vi "Read Available Data Names.vi"(8 "error in (no error)":errorcluster, 11 "ControlDropMsg in":refnum<class "ControlDropMsg.lvclass">) -> (0 "error out":errorcluster, 2 "Available Data Names":string[](array[string]), 3 "ControlDropMsg out":refnum<class "ControlDropMsg.lvclass">)   [LabVIEW 2017, in "ActorEvents.lvlib" / "ControlDropMsg.lvclass"]
uses:
  ControlDropMsg.lvclass
  ControlDropMsg.lvclass/ControlDropMsg.ctl
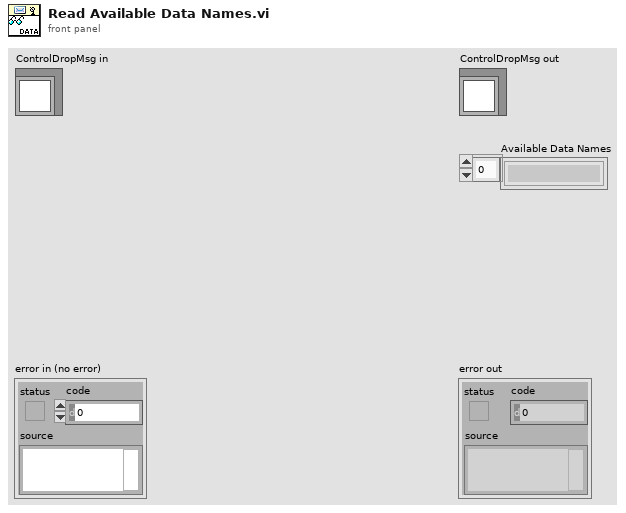
[diagram p1: front panel]
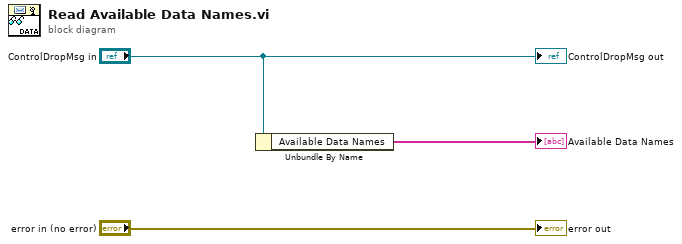
[diagram p0: block diagram]
diagram:
  n1 = Unbundle By Name("ControlDropMsg in") -> ("Available Data Names"=→"Available Data Names":string[])
  "error out" <- "error in (no error)"
  "ControlDropMsg out" <- "ControlDropMsg in"
